vi "main screen.vi"() -> ()   [LabVIEW 2020]
uses:
  <vilib>/DAQmx/read.llb/DAQmx Read (Analog 1D DBL NChan 1Samp).vi
  <vilib>/DAQmx/configure/timing.llb/DAQmx Timing (Sample Clock).vi
  <vilib>/vision/driver/NI_Vision_Acquisition_Software.lvlib
  <vilib>/userdefined/High Color/IMAQdx.ctl
  <resource>/objmgr/imaqdx.rc
  <vilib>/DAQmx/create/channels.llb/DAQmx Create Channel (AI-Voltage-Basic).vi
  <vilib>/DAQmx/create/channels.llb/DAQmx Create Channel (AI-Temperature-Thermocouple).vi
  <vilib>/DAQmx/create/channels.llb/DAQmx Create Channel (DO-Digital Output).vi
  <vilib>/DAQmx/write.llb/DAQmx Write (Digital Bool 1Line 1Point).vi
  <vilib>/vision/NI_Vision_Development_Module.lvlib
panel:
  in  "laser on\\off":bool
  in  "stop":bool
  in  "physical channels":tag
  in  "TC channel":tag
  out "Image 2":T1(plugin-control)
  out "Image":T1(plugin-control)
  out "T.C 8":dbl[](graph)
  out "System Time (s)":dbl
  out "T.C 1":dbl[](graph)
  out "Rear Diode":dbl[](graph)
  out "Front Diode":dbl[](graph)
  out "T.C 7":dbl[](graph)
  out "T.C 6":dbl[](graph)
  out "T.C 5":dbl[](graph)
  out "T.C 4":dbl[](graph)
  out "T.C 3":dbl[](graph)
  out "T.C 2":dbl[](graph)
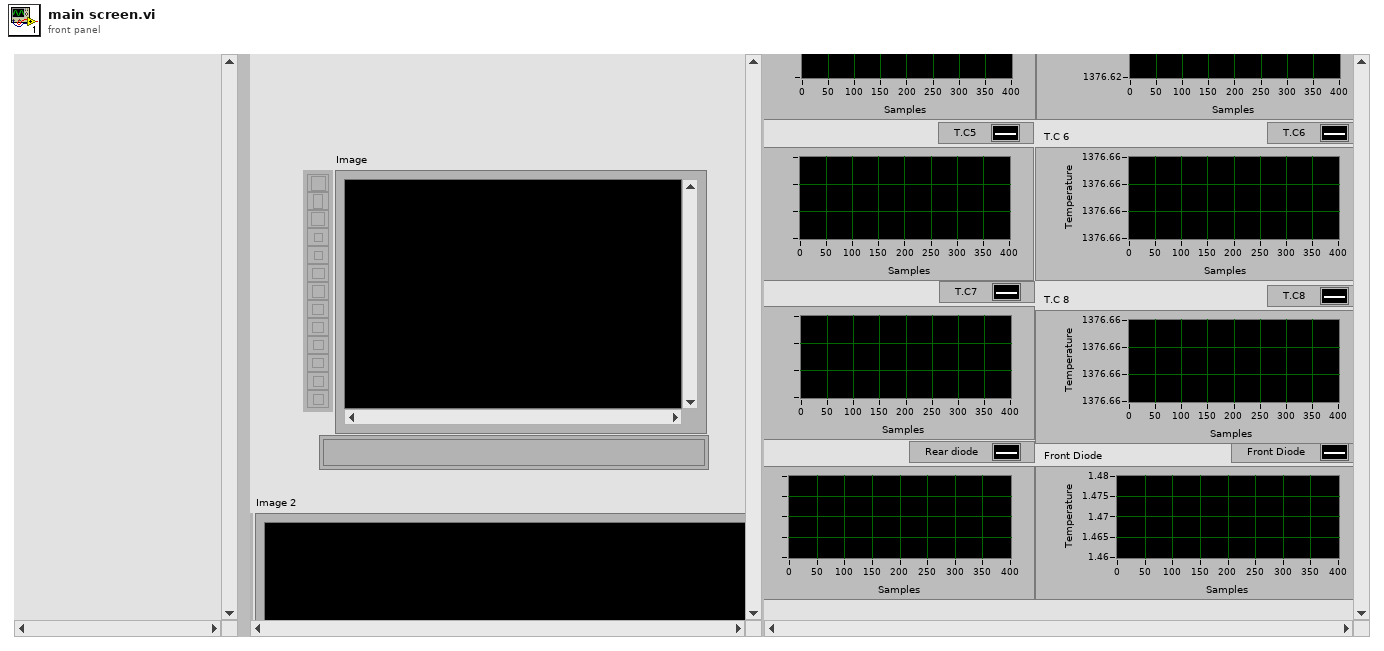
[diagram p1: front panel]
types:
  T1 = typedef "IMAQ Image.ctl" = refnum<image>
  T2 = typedef "IMAQdx.ctl" = refnum<k21>
  T3 = typedef "IMAQ AVI2 Refnum.ctl" = refnum<k20>
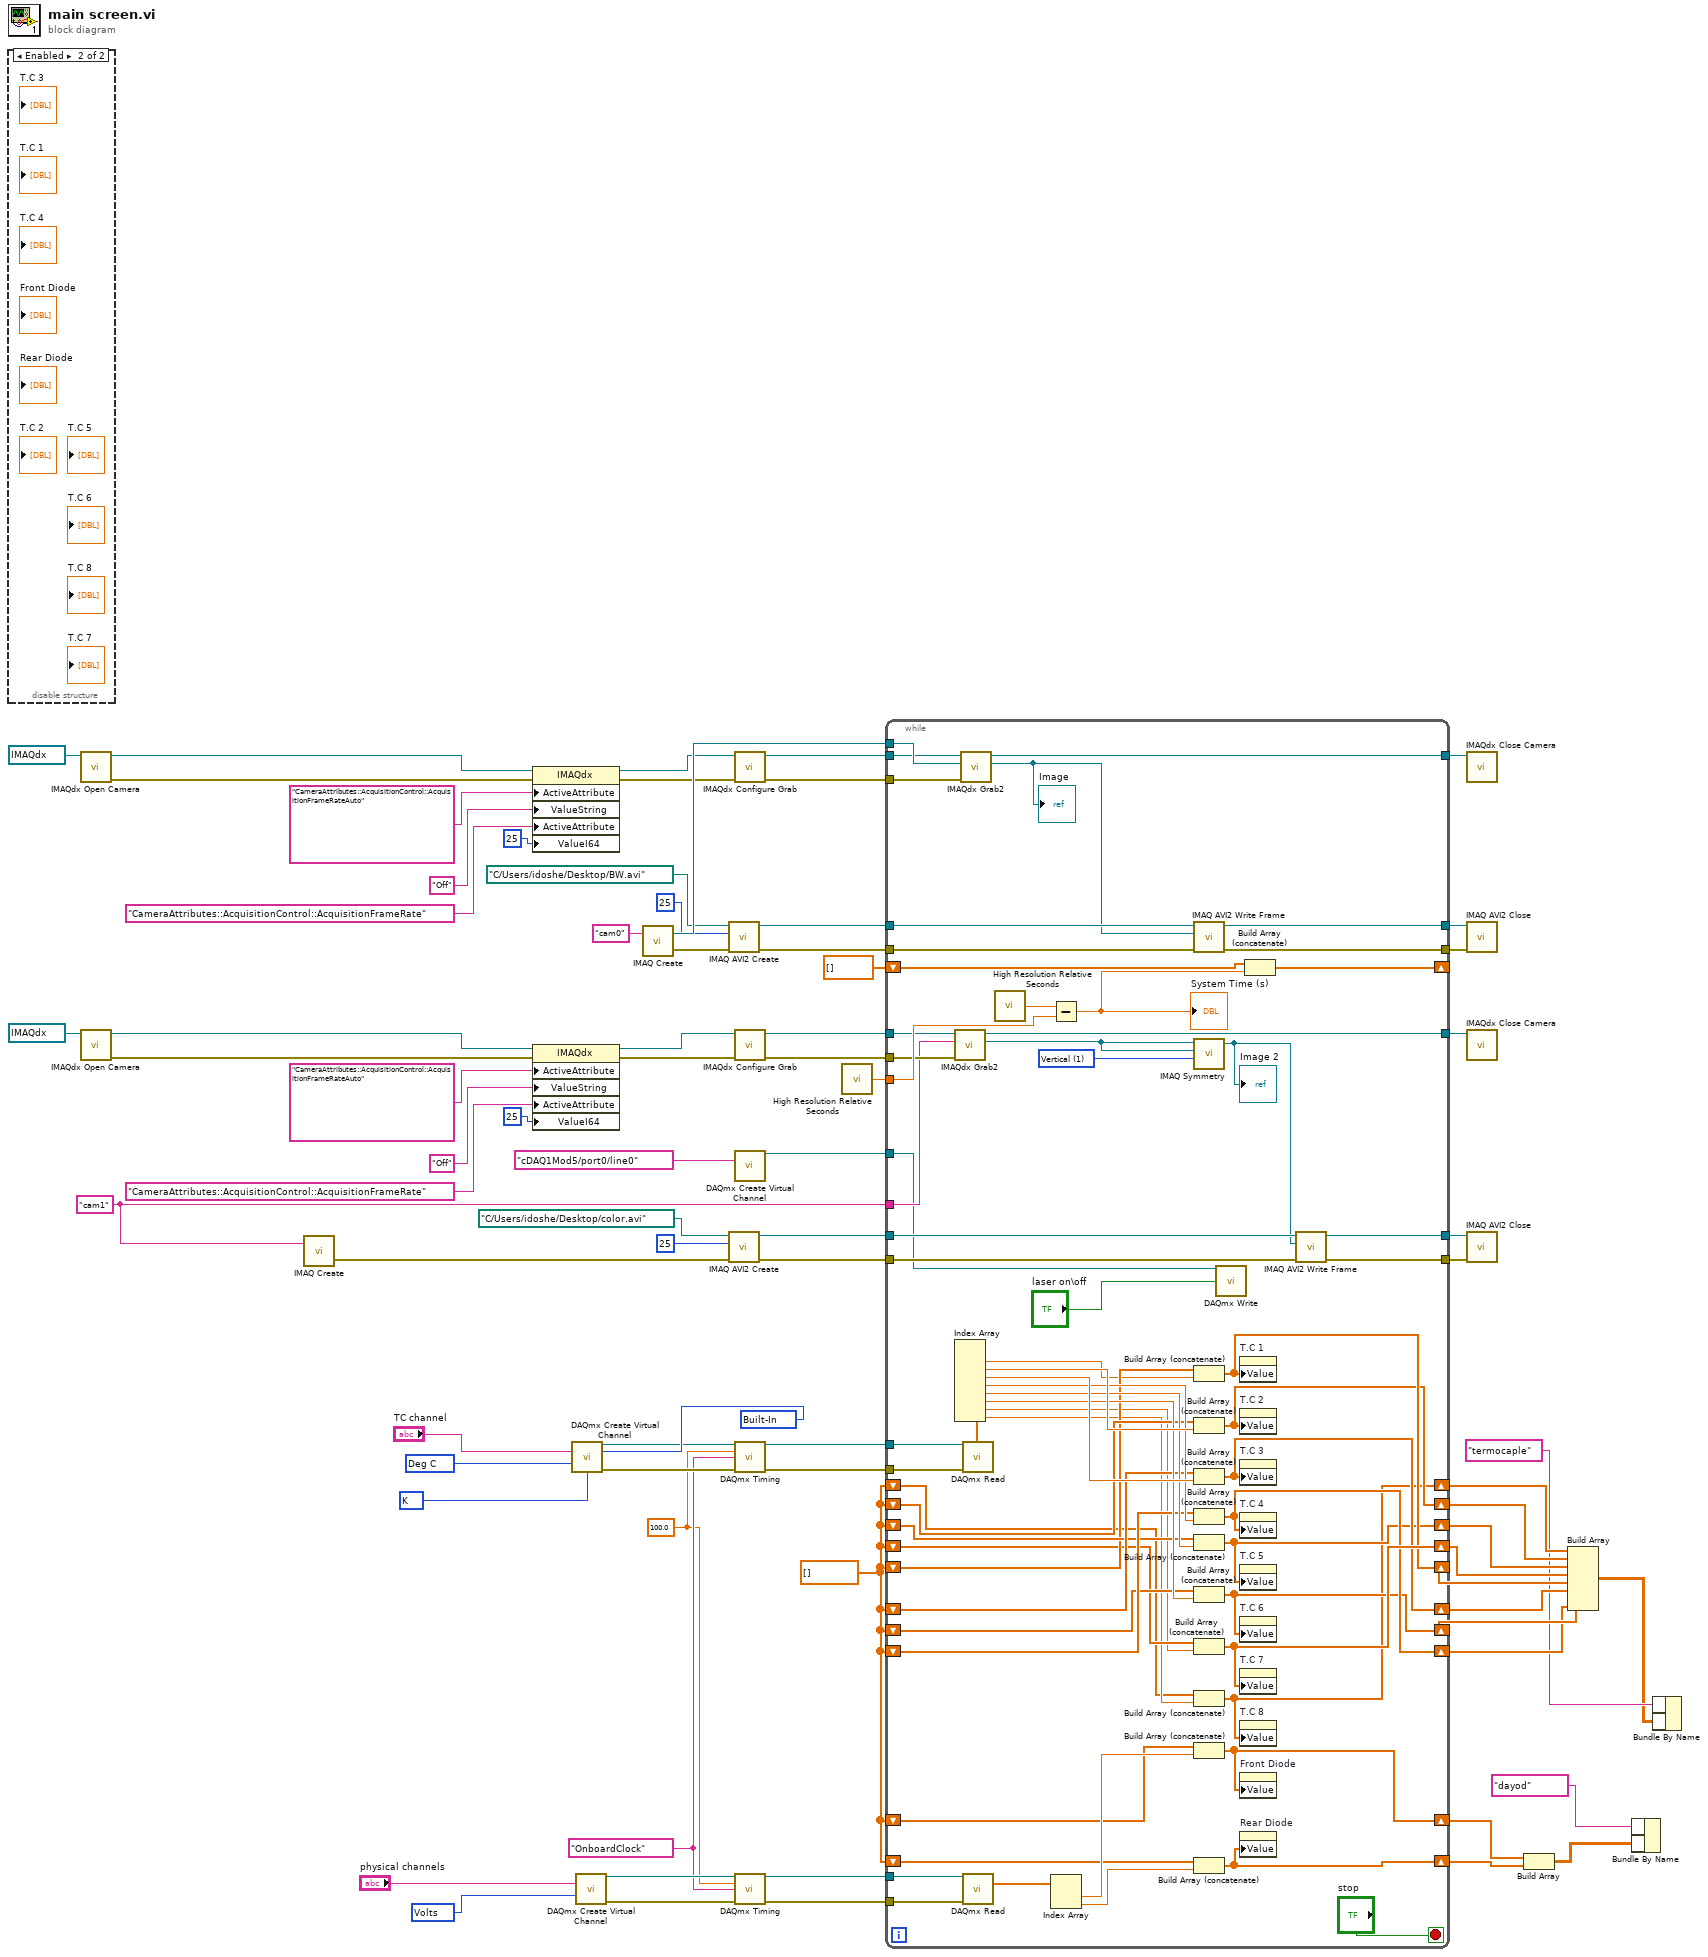
[diagram p0: block diagram]
diagram:
  w15 = 10073 items=["J"=10072, "K"=10073, "N"=10077, "R"=10082, "S"=10085, "T"=10086, "B"=10047, "E"=10055] ("thermocouple type")
  w35 = "cam1" ("Image Name")
  w65 = 100.0 ("rate")
  w66 = tag "OnboardClock" ("source")
  w72 = 10348 items=["Volts"=10348, "From Custom Scale"=10065] ("units")
  w18 = dbl[] []
  w74 = 10200 items=["Built-In"=10200, "Constant Value"=10116, "Channel"=10113] ("cjc source")
  w75 = 10143 items=["Deg C"=10143, "Deg F"=10144, "Kelvins"=10325, "Deg R"=10145, "From Custom Scale"=10065] ("units")
  n1 = disable-structure shown="Enabled" {
    frame Disabled {
    }
    frame Enabled {
    }
  }
  n2 = call <vilib>:"IMAQdx Open Camera.vi"("Session In"=T2 "cam0") -> ("error out"=w51:errorcluster, "Session Out"=w53:T2)  [unwired: 9 in]
  n3 = call <vilib>:"IMAQdx Open Camera.vi"("Session In"=T2 "cam1") -> ("error out"=w42:errorcluster, "Session Out"=w44:T2)  [unwired: 9 in]
  n4 = call "IMAQ Create"("Image Name"=w35) -> ("error out"=w32:errorcluster)  [unwired: 4 in, 1 out]
  n5 = property class="IMAQdx"(reference=w53, error in=w51, "ActiveAttribute"="CameraAttributes::AcquisitionControl::AcquisitionFrameRateAuto", "ValueString"="Off", "ActiveAttribute"="CameraAttributes::AcquisitionControl::AcquisitionFrameRate", "ValueI64"=u32 25 ("ValueU32")) -> (reference out=w52:T2, error out=w50:errorcluster)
  n6 = property class="IMAQdx"(reference=w44, error in=w42, "ActiveAttribute"="CameraAttributes::AcquisitionControl::AcquisitionFrameRateAuto", "ValueString"="Off", "ActiveAttribute"="CameraAttributes::AcquisitionControl::AcquisitionFrameRate", "ValueI64"=u32 25 ("ValueU32")) -> (reference out=w43:T2, error out=w41:errorcluster)
  n7 = call-poly <vilib>:"DAQmx Create Virtual Channel.vi"("physical channels"="TC channel", "cjc source"=w74, "units"=w75, "thermocouple type"=w15) -> ("task out"=w68:refnum<k21>, "error out"=w67:errorcluster)  [unwired: 10 in]
  n8 = call-poly <vilib>:"DAQmx Create Virtual Channel.vi"("physical channels"="physical channels", "units"=w72) -> ("task out"=w71:refnum<k21>, "error out"=w70:errorcluster)  [unwired: 12 in]
  n9 = call "IMAQ Create"("Image Name"="cam0") -> ("New Image"=w57:T1, "error out"=w25:errorcluster)  [unwired: 4 in]
  n10 = call "IMAQ AVI2 Create"("error in (no error)"=w25, "Frames Per Second"=u32 25, "AVI Path"=path "C:/Users/idoshe/Desktop/BW.avi") -> ("error out"=w21:errorcluster, "AVI Refnum"=w22:T3)  [unwired: 7 in]
  n11 = call "IMAQ AVI2 Create"("error in (no error)"=w32, "Frames Per Second"=u32 25, "AVI Path"=path "C:/Users/idoshe/Desktop/color.avi") -> ("error out"=w30:errorcluster, "AVI Refnum"=w31:T3)  [unwired: 7 in]
  n12 = call <vilib>:"IMAQdx Configure Grab.vi"("error in"=w50, "Session In"=w52) -> ("error out"=w58:errorcluster, "Session Out"=w56:T2)  [unwired: 8 in]
  n13 = call <vilib>:"IMAQdx Configure Grab.vi"("error in"=w41, "Session In"=w43) -> ("error out"=w26:errorcluster, "Session Out"=w27:T2)  [unwired: 8 in]
  n14 = call-poly <vilib>:"DAQmx Create Virtual Channel.vi"("lines"=tag "cDAQ1Mod5/port0/line0") -> ("task out"=w16:refnum<k21>)  [unwired: 13 in, 1 out]
  n15 = call-poly <vilib>:"DAQmx Timing.vi"("task/channels in"=w68, "rate"=w65, "source"=w66, "error in"=w67) -> ("task out"=w63:refnum<k21>, "error out"=w64:errorcluster)  [unwired: 10 in]
  n16 = call-poly <vilib>:"DAQmx Timing.vi"("task/channels in"=w71, "rate"=w65, "source"=w66, "error in"=w70) -> ("task out"=w69:refnum<k21>, "error out"=w62:errorcluster)  [unwired: 10 in]
  n17 = call <vilib>:"High Resolution Relative Seconds.vi"() -> ("relative seconds"=w61:dbl)
  n18 = while {
    tunnel: w63 -> [w140]
    tunnel: w64 -> [w139]
    shift-right: [w123] -> w13
    shift-left: w18 -> [w132]
    shift-right: [w122] -> w9
    shift-left: w18 -> [w131]
    shift-right: [w121] -> w7
    shift-left: w18 -> [w130]
    shift-right: [w120] -> w12
    shift-left: w18 -> [w129]
    shift-right: [w119] -> w8
    shift-left: w18 -> [w128]
    shift-right: [w124] -> w10
    shift-left: w18 -> [w127]
    shift-right: [w125] -> w11
    shift-left: w18 -> [w126]
    tunnel: w69 -> [w118]
    tunnel: w62 -> [w117]
    shift-right: [w113] -> w6
    shift-left: w18 -> [w114]
    shift-right: [w110] -> w5
    shift-left: w18 -> [w111]
    tunnel: w61 -> [w109]
    shift-right: [w106] -> _
    shift-left: dbl[] [] -> [w105]
    shift-right: [w100] -> w14
    shift-left: w18 -> [w101]
    tunnel: w58 -> [w99]
    tunnel: w57 -> [w98]
    tunnel: w56 -> [w97]
    tunnel: [w96] -> w55
    tunnel: w27 -> [w94]
    tunnel: w26 -> [w93]
    tunnel: [w92] -> w36
    tunnel: w35 -> [w91]
    tunnel: w31 -> [w90]
    tunnel: w30 -> [w89]
    tunnel: [w88] -> w29
    tunnel: [w87] -> w28
    tunnel: w22 -> [w86]
    tunnel: w21 -> [w85]
    tunnel: [w83] -> w20
    tunnel: [w82] -> w19
    tunnel: w16 -> [w81]
    stop <- "stop" stop-if-true
    w79 = u32 1 items=["Horizontal", "Vertical", "Central", "1st Diagonal", "2nd Diagonal"] ("Type of Symmetry")
    n19 = call <vilib>:"IMAQdx Grab2.vi"("error in"=w93, "Image In"=w91, "Session In"=w94) -> ("Image Out"=w78:T1, "Session Out"=w92:T2)  [unwired: 5 in, 2 out]
    n20 = call <vilib>:"IMAQdx Grab2.vi"("error in"=w99, "Image In"=w98, "Session In"=w97) -> ("Image Out"=w84:T1, "Session Out"=w96:T2)  [unwired: 5 in, 2 out]
    "Image" <- w84
    n21 = call-poly <vilib>:"DAQmx Read.vi"("task/channels in"=w140, "error in"=w139) -> ("data"=w138:dbl[])  [unwired: 11 in, 2 out]
    n22 = Index Array(array=w138) -> (element #1=w104:dbl, element #2=w137:dbl, element #3=w136:dbl, element #4=w135:dbl, element #5=w134:dbl, element #6=w133:dbl, element #7=w103:dbl, element #8=w102:dbl)  [unwired: 8 in]
    n23 = call-poly <vilib>:"DAQmx Read.vi"("task/channels in"=w118, "error in"=w117) -> ("data"=w116:dbl[])  [unwired: 11 in, 2 out]
    n24 = call <vilib>:"High Resolution Relative Seconds.vi"() -> ("relative seconds"=w108:dbl)
    n25 = Subtract(x=w108, y=w109) -> (x-y=w107:dbl)
    "System Time (s)" <- w107
    n26 = Index Array(array=w116) -> (element #1=w115:dbl, element #2=w112:dbl)  [unwired: 2 in]
    n27 = call "IMAQ AVI2 Write Frame"("error in (no error)"=w85, "Image"=w84, "AVI Refnum"=w86) -> ("error out"=w82:errorcluster, "AVI Refnum (duplicate)"=w83:T3)  [unwired: 6 in, 1 out]
    n28 = call "IMAQ Symmetry"("Type of Symmetry"=w79, "Image Dst"=w78, "Image Src"=w78) -> ("Image Dst Out"=w77:T1)  [unwired: 2 in, 1 out]
    "Image 2" <- w77
    n29 = Build Array (concatenate)(w127, w104) -> (w124:dbl[])
    n30 = Build Array (concatenate)(w132, w137) -> (w123:dbl[])
    n31 = Build Array (concatenate)(w131, w136) -> (w122:dbl[])
    n32 = Build Array (concatenate)(w130, w135) -> (w121:dbl[])
    n33 = Build Array (concatenate)(w129, w134) -> (w120:dbl[])
    n34 = Build Array (concatenate)(w128, w133) -> (w119:dbl[])
    n35 = Build Array (concatenate)(w126, w103) -> (w125:dbl[])
    n36 = Build Array (concatenate)(w101, w102) -> (w100:dbl[])
    n37 = Build Array (concatenate)(w114, w115) -> (w113:dbl[])
    n38 = Build Array (concatenate)(w111, w112) -> (w110:dbl[])
    n39 = call-poly <vilib>:"DAQmx Write.vi"("task/channels in"=w81, "data"="laser on\\off") -> ()  [unwired: 11 in, 3 out]
    n40 = property on="T.C 1" class="WFGraph (strict)"("Value"=w124) -> ()  [unwired: 2 in, 2 out]
    n41 = property on="T.C 2" class="WFGraph (strict)"("Value"=w123) -> ()  [unwired: 2 in, 2 out]
    n42 = property on="T.C 3" class="WFGraph (strict)"("Value"=w122) -> ()  [unwired: 2 in, 2 out]
    n43 = property on="T.C 4" class="WFGraph (strict)"("Value"=w121) -> ()  [unwired: 2 in, 2 out]
    n44 = property on="T.C 5" class="WFGraph (strict)"("Value"=w120) -> ()  [unwired: 2 in, 2 out]
    n45 = property on="T.C 6" class="WFGraph (strict)"("Value"=w119) -> ()  [unwired: 2 in, 2 out]
    n46 = property on="T.C 7" class="WFGraph (strict)"("Value"=w125) -> ()  [unwired: 2 in, 2 out]
    n47 = property on="T.C 8" class="WFGraph (strict)"("Value"=w100) -> ()  [unwired: 2 in, 2 out]
    n48 = property on="Front Diode" class="WFGraph (strict)"("Value"=w113) -> ()  [unwired: 2 in, 2 out]
    n49 = property on="Rear Diode" class="WFGraph (strict)"("Value"=w110) -> ()  [unwired: 2 in, 2 out]
    n50 = Build Array (concatenate)(w105, w107) -> (w106:dbl[])
    n51 = call "IMAQ AVI2 Write Frame"("error in (no error)"=w89, "Image"=w77, "AVI Refnum"=w90) -> ("error out"=w87:errorcluster, "AVI Refnum (duplicate)"=w88:T3)  [unwired: 6 in, 1 out]
  }
  n52 = call <vilib>:"IMAQdx Close Camera.vi"("Session In"=w55) -> ()  [unwired: 10 in, 1 out]
  n53 = call "IMAQ AVI2 Close"("error in (no error)"=w19, "AVI Refnum"=w20) -> ()  [unwired: 9 in, 1 out]
  n54 = call <vilib>:"IMAQdx Close Camera.vi"("Session In"=w36) -> ()  [unwired: 10 in, 1 out]
  n55 = call "IMAQ AVI2 Close"("error in (no error)"=w28, "AVI Refnum"=w29) -> ()  [unwired: 9 in, 1 out]
  n56 = Build Array(w6, w5) -> (w2:dbl[][])
  n57 = Build Array(w14, w13, w12, w11, w10, w9, w8, w7) -> (w1:dbl[][])
  n58 = Bundle By Name("dayod", w2) -> ()  [unwired: 1 in, 1 out]
  n59 = Bundle By Name("termocaple", w1) -> ()  [unwired: 1 in, 1 out]
